vi "DETECTFIRSTBALL.vi"   [LabVIEW 2016, in "Test2.lvrbt"]
uses:
  Test2.lvrbt
  <vilib>/NXT/Block Support/NXT_InputPort.ctl
  <vilib>/NXT/Hardware/Plugins/Tetrix DC Motor/TetrixDCMotorAddress.ctl
  <vilib>/NXT/Hardware/Plugins/Tetrix 180 deg Servo/Tetrix180ServoAddress.ctl
  <vilib>/NXT/NXTIO Xnodes/NXTIONodeSubVIs/TETRIX IO Move Servos.vi
  <vilib>/NXT/Dual Mode Library/Waits/Wait_Num.vi
  <vilib>/NXT/NXTIO Xnodes/NXTIONodeSubVIs/TETRIX IO Move DC Motors.vi
  <vilib>/NXT/Dual Mode Library/Waits/Wait_EV3_Ultrasonic_Centimeters_Further.vi
  <vilib>/NXT/NXTIO Xnodes/NXTIONodeSubVIs/TETRIX IO Stop DC Motors.vi
  <vilib>/NXT/Dual Mode Library/Waits/Wait_EV3_Ultrasonic_Centimeter_Closer.vi
  <vilib>/NXT/NXTIO Xnodes/AddressXNode/NXTIOAddress.xnode
  <vilib>/NXT/Subs/LVHSConnector.ctl
  <vilib>/NXT/NXTIO Xnodes/NXTIOXNode/NXTIO.xnode
  <vilib>/NXT/LegoClasses/BrickReference/BrickReference.lvclass
types:
  T1 = typedef "NXT_InputPort.ctl" = u32
  T2 = typedef "Tetrix180ServoAddress.ctl" = i32
  T3 = cluster{"Tetrix180Servo":T2, "Tetrix180Servo":T2, "Tetrix180Servo":T2, "Tetrix180Servo":T2, "Tetrix180Servo":T2, "Tetrix180Servo":T2}
  T4 = typedef "LVHSConnector.ctl" = refnum<class "BrickReference.lvclass">
  T5 = typedef "TetrixDCMotorAddress.ctl" = i32
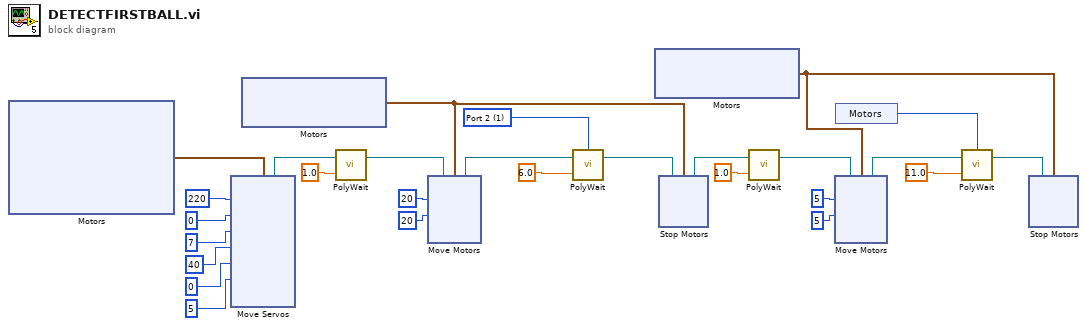
[diagram p0: block diagram]
diagram:
  w23 = T1 1 items=["Port 1", "Port 2", "Port 3", "Port 4"] ("Port (Port 1)")
  n1 = xnode "Motors"() -> ("Motor"=w18:T3)
  n2 = xnode "Move Servos"("Position 6"=u8 5, "Position 5"=u8 0, "Position 4"=u8 40, "Position 3"=u8 7, "Position 2"=u8 0, "Position 1"=u8 220, "Motors"=w18) -> ("NXT/EV3"=w11:T4)  [unwired: 1 in]
  n3 = xnode "Motors"() -> ("Motor"=w19:cluster{"TetrixDCMotor":T5, "TetrixDCMotor":T5})
  n4 = call-poly <vilib>:"PolyWait.vi"("Time (1 sec)"=sgl 1.0, "NXT/EV3"=w11) -> ("NXT/EV3"=w20:T4)  [unwired: 2 in]
  n5 = xnode "Move Motors"("Power/Speed 2"=i8 20, "Power/Speed 1"=i8 20, "Motors"=w19, "NXT/EV3"=w20) -> ("NXT/EV3"=w26:T4)
  n6 = call-poly <vilib>:"PolyWait.vi"("Centimeters (50)"=sgl 6.0, "NXT/EV3"=w26, "Port (Port 1)"=w23) -> ("NXT/EV3"=w24:T4)  [unwired: 1 in]
  n7 = xnode "Motors"() -> ("Motor"=w7:cluster{"TetrixDCMotor":T5, "TetrixDCMotor":T5})
  n8 = xnode "Stop Motors"("Motors"=w19, "NXT/EV3"=w24) -> ("NXT/EV3"=w1:T4)
  n9 = call-poly <vilib>:"PolyWait.vi"("Time (1 sec)"=sgl 1.0, "NXT/EV3"=w1) -> ("NXT/EV3"=w2:T4)  [unwired: 2 in]
  n10 = xnode "Move Motors"("Power/Speed 2"=i8 5, "Power/Speed 1"=i8 5, "Motors"=w7, "NXT/EV3"=w2) -> ("NXT/EV3"=w9:T4)
  n11 = xnode "Motors"() -> ("Sensor"=w4:T1)
  n12 = call-poly <vilib>:"PolyWait.vi"("Centimeters (40)"=sgl 11.0 ("Centimeters (50)"), "NXT/EV3"=w9, "Port (Port 1)"=w4) -> ("NXT/EV3"=w8:T4)  [unwired: 1 in]
  n13 = xnode "Stop Motors"("Motors"=w7, "NXT/EV3"=w8) -> ()  [unwired: 1 out]
